vi "Controls - By Folder.vi"(7 "Msg Chain":string, 8 "error in (no error)":errorcluster {"code" format="Error %.0f"}, 10 "Controls Docs":refnum<class "GUI Documentation.lvclass">[](array[class]), 11 "VIDoc Printer - Confluence In":refnum<class "VIDoc Printer - Confluence.lvclass">) -> (0 "error out":errorcluster {"code" format="Error %.0f"}, 3 "VIDoc Printer - Confluence Out":refnum<class "VIDoc Printer - Confluence.lvclass">)   [LabVIEW 2023, in "VIDoc Printer - Confluence.lvlib" / "VIDoc Printer - Confluence.lvclass"]
uses:
  VIDoc Printer - Confluence.lvclass
  Parsing/GUI Documentation/GUI Documentation.lvclass
  Confluence Formatting/Types/Format Combo Box.ctl
  VIDoc Printer - Confluence.lvclass/VIDoc Printer - Confluence.ctl
  Parsing/GUI Documentation/GUI Documentation.lvclass/GUI Documentation.ctl
  Parsing/GUI Documentation/Get VI Info.vi
  Accessors/Get Ctrls By Folder Expand.vi
  Confluence Formatting/Confluence Formatting.lvlib
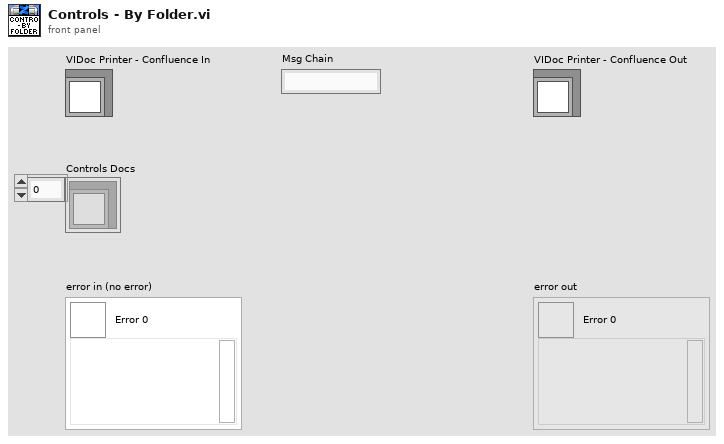
[diagram p1: front panel]
types:
  T1 = typedef "Confluence Formatting.lvlib/Format Combo Box.ctl" = string
  T2 = typedef "VIDoc Parsing.lvlib/Method Spec Cluster.ctl" = cluster{"VI Type Ext":T3, "Name":string, "Path":path, "Get Conpane Image":T4, "Description":string, "Get Library Access Scope":enum32{"invalid scope", "public", "private", "protected", "community"}, "Dispatch":T5, "ContainsCompiledCode":bool, "Exec.IsReentrant":bool, "Exec.ReentrancyType":enum16{"Share clones between instances", "Preallocate clone for each instance"}, "ExecInlining":bool, "ExecInlineIfPossible":bool, "Auto Err Handling":bool, "CodeComplexity":sgl, "Bookmark Tags":string[], "Control VI Type":enum32{"not a control VI", "control", "typedef", "strict typedef"}, "Controls":T6[], "VI Type":enum32{"invalid VI type", "Standard VI", "Control VI", "Global VI", "Polymorphic VI", "Configuration VI", "SubSystem", "Facade VI", "Method VI", "Statechart Diagram VI"}, "Minimum Size":T8, "Front Panel Window:Title":string, "Front Panel Window:Behavior":enum32{"Invalid", "Default", "Floating", "Floating/Auto-Hide", "Modal"}, "Front Panel Window:Closeable":bool, "Must Override":bool, "Must Use Parent Implementation":bool, "VI Icon":T4, "Front Panel":T4, "History:Revision Number":u32, "Metrics:Total Data Size":u32, "Execution:Allow Debugging":bool, "Execution:Preferred Exec System":enum32{"invalid execution system", "user interface", "standard", "instrument i/o", "data acquisition", "other 1", "other 2", "same as caller"}, "Execution:Priority":enum32{"invalid priority", "background priority", "normal priority", "above normal priority", "high priority", "time critical priority", "subroutine"}, "BM Tag Text":string[], "Block Diagram":T4, "Structure Tree":T9[]}
  T3 = typedef "VIDoc Parsing.lvlib/VI Type Extended Enum.ctl" = enum16{"Unknown", "Class Method", "Class Accessor Get", "Class Accessor Set", "Class Control", "Library Method", "Library Control", "VI", "Control"}
  T4 = typedef "imagedata.ctl" = cluster{"image type":i32, "image depth":i32, "image":u8[], "mask":u8[], "colors":u32[], "Rectangle":cluster{"left":i16, "top":i16, "right":i16, "bottom":i16}}
  T5 = typedef "VIDoc Parsing.lvlib/Class Dispatch Type Enum.ctl" = enum16{"None", "Static", "Dynamic"}
  T6 = typedef "VIDoc Parsing.lvlib/Controls Info Cluster.ctl" = cluster{"Name":string, "Description":string, "Data Type":string, "Tip Strip":string, "UID":i32, "Image Data":T4, "ToggleKeyBind":T7, "Raw Label":string, "Raw Caption":string}
  T7 = typedef "LVKeyTypeDef.ctl" = cluster{"Focus":bool, "Control":bool, "Shift":bool, "Key":string}
  T8 = typedef "LVPointTypeDef.ctl" = cluster{"Horizontal":i16, "Vertical":i16}
  T9 = typedef "VIDoc Parsing.lvlib/Structure Reporter.lvlib/Tree Cluster.ctl" = cluster{"Object Class Name":string, "Labels":string[], "Child Tag":string, "Item Indent":i32, "Child Only?":bool, "Glyph Index":i32}
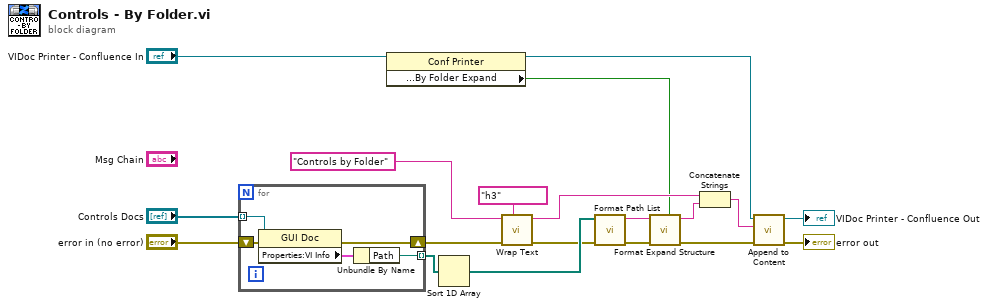
[diagram p0: block diagram]
diagram:
  n1 = for {
    tunnel: "Controls Docs" -> [w23] mode=indexing
    tunnel: [w20] -> w18 mode=indexing
    shift-right: [w21] -> w17
    shift-left: "error in (no error)" -> [w24]
    n2 = property class="GUI Doc"(reference=w23, error in=w24) -> (error out=w21:errorcluster, "Properties:VI Info"=w22:T2)  [unwired: 1 out]
    n3 = Unbundle By Name(w22) -> ("Path"=w20:path)
  }
  n4 = property class="Conf Printer"(reference="VIDoc Printer - Confluence In") -> (reference out=w2:refnum<class "VIDoc Printer - Confluence.lvclass">, "Properties:Expand?:Control:By Folder Expand"=w1:bool)  [unwired: 1 in, 1 out]
  n5 = Sort 1D Array(array=w18) -> (sorted array=w14:path[])
  n6 = call "Wrap Text.vi"("Formatting"=T1 "h3", "Error in"=w17, "String"="Controls by Folder" ("format string")) -> ("Error out"=w13:errorcluster, "Wrapped String"=w16:string)  [unwired: 7 in]
  n7 = call "Format Path List.vi"("Error in"=w13, "Paths"=w14) -> ("Error out"=w12:errorcluster, "Bullet List String"=w4:string)  [unwired: 8 in]
  n8 = call "Format Expand Structure.vi"("Enable? (T)"=w1, "Error in"=w12, "Content"=w4) -> ("Error out"=w5:errorcluster, "Expand String"=w3:string)  [unwired: 7 in]
  n9 = Concatenate Strings(w16, w3) -> (w15:string)
  n10 = call "Append to Content.vi"("error in (no error)"=w5, "Content"=w15, "VIDoc Printer - Confluence In"=w2) -> ("error out"=→"error out":errorcluster, "VIDoc Printer - Confluence Out"=→"VIDoc Printer - Confluence Out":refnum<class "VIDoc Printer - Confluence.lvclass">)  [unwired: 7 in]
